vi "Set String Value.vi"(0 "No Error":string, 1 "String to Format (not a refnum)":refnum<vi>) -> ()   [LabVIEW 2020]
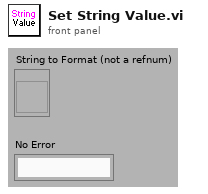
[diagram p1: front panel]
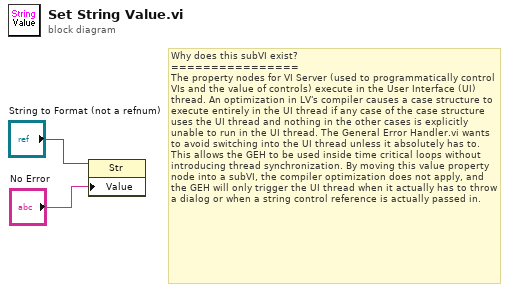
[diagram p0: block diagram]
diagram:
  # "Why does this subVI exist?\n================\nThe property nodes for VI Server (used to programmatically control VIs and the value of controls) execute in the User Interface (UI) thread. An optimization in LV's compiler causes a case structure to execute entirely in the UI thread if any case of the case structure uses the UI thread and nothing in the other cases is explicitly unable to run in the UI thread. The General Error Handler.vi wants to avoid switching into the UI thread unless it absolutely has to. This allows the GEH to be used inside time critical loops without introducing thread synchronization. By moving this value property node into a subVI, the compiler optimization does not apply, and the GEH will only trigger the UI thread when it actually has to throw a dialog or when a string control reference is actually passed in."
  n1 = property class="Str"(reference="String to Format (not a refnum)", "Value"="No Error") -> ()  [unwired: 1 in, 2 out]
